vi "sortAndQueueLines.vi"(7 "scanning?":bool, 8 "error in (no error)":errorcluster, 11 "Queues":T2) -> (0 "error out":errorcluster, 1 "lost vol":cluster{"volume num":u32, "volume num":u32}[](array[cluster]), 3 "stats":T1, 5 "not waiting for new lines":bool)   [LabVIEW 2010]
uses:
  internal_queues.ctl
  line_info.ctl
  volume_with_lines.ctl
  volume_info.ctl
  kalman_result_scaled.ctl
  location3D.ctl
  spot location.ctl
  splitLinesIntoVolumes.vi
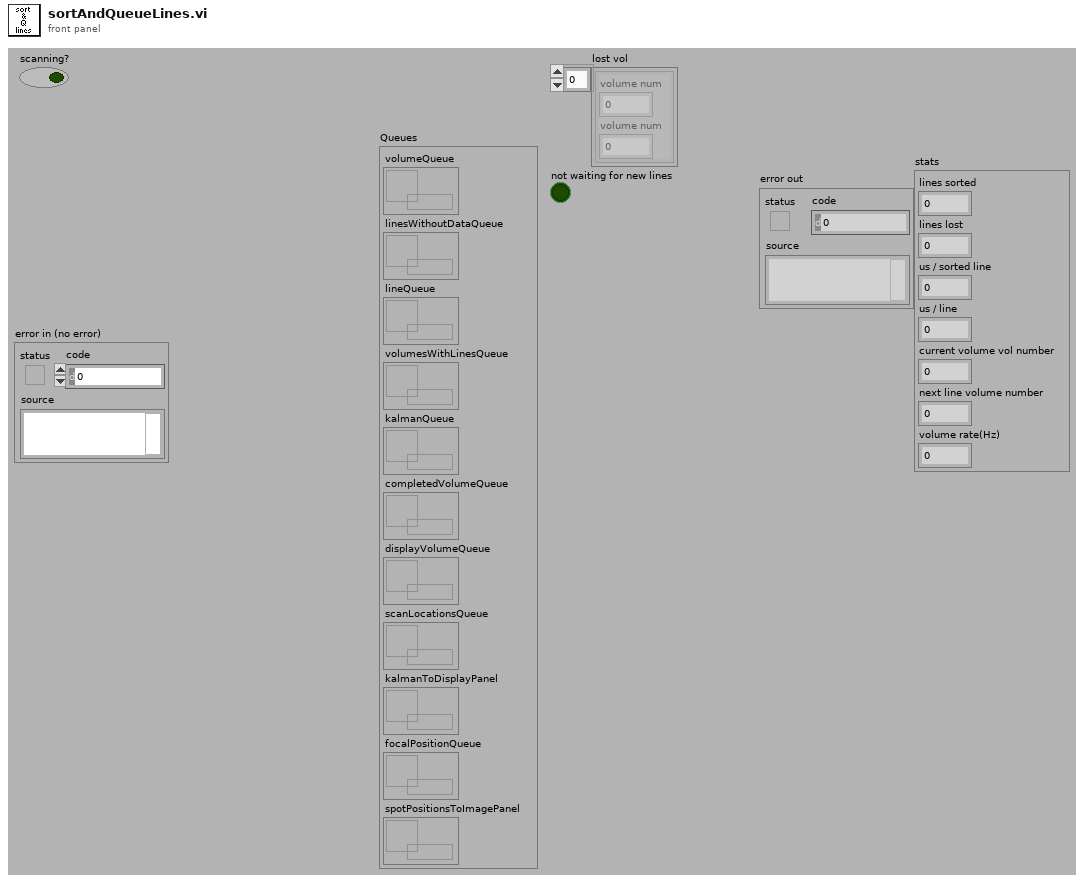
[diagram p1: front panel]
types:
  T1 = cluster{"lines sorted":i32, "lines lost":i32, "us / sorted line":dbl, "us / line":dbl, "current volume vol number":u32, "next line volume number":u32, "volume rate(Hz)":dbl}
  T2 = typedef "internal_queues.ctl" = cluster{"volumeQueue":refnum<queue>, "linesWithoutDataQueue":refnum<queue>, "lineQueue":refnum<queue>, "volumesWithLinesQueue":refnum<queue>, "kalmanQueue":refnum<queue>, "completedVolumeQueue":refnum<queue>, "displayVolumeQueue":refnum<queue>, "scanLocationsQueue":refnum<queue>, "kalmanToDisplayPanel":refnum<queue>, "focalPositionQueue":refnum<queue>, "spotPositionsToImagePanel":refnum<queue>}
  T3 = typedef "line_info.ctl" = cluster{"start X":i16, "start Y":i16, "start Z":i16, "end X":i16, "end Y":i16, "end Z":i16, "num z":u8, "voxel data":u32[], "volume num":u32, "line number":u16, "line type":u16}
  T4 = cluster{i32, i32, dbl, dbl, "last volume processed":u32, "volume num":u32, dbl}
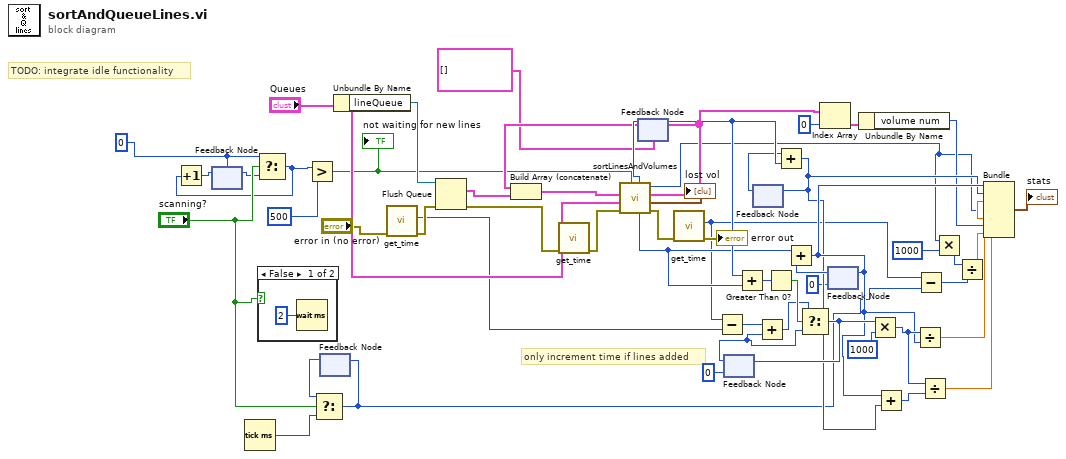
[diagram p0: block diagram]
diagram:
  w4 = u32 0 ("t")
  # "TODO: integrate idle functionality"
  # "only increment time if lines added"
  n1 = feedback #1(w4) -> (w5:u32)
  n2 = Tick Count (ms)() -> (millisecond timer value=w18:u32)
  n3 = Select(t=w4, s="scanning?", f=w5) -> (s? t:f=w3:u32)
  n4 = Increment(x=w3) -> (x+1=w6:u32)
  n5 = feedback-in #1(w6) -> ()
  n6 = case shown="False" "scanning?" {
    frame False {
      n7 = Wait (ms)(milliseconds to wait=u32 2) -> ()  [unwired: 1 out]
    }
    frame True {
    }
  }
  n8 = Greater?(x=w3, y=u32 500) -> (0:w1:bool)
  "not waiting for new lines" <- w1
  n9 = feedback #2() -> (w17:u32)  [unwired: 1 in]
  n10 = Select(t=w17, s="scanning?", f=w18) -> (s? t:f=w15:u32)
  n11 = feedback-in #2(w15) -> ()
  n12 = Unbundle By Name("Queues") -> ("lineQueue"=w54:refnum<queue>)
  n13 = call "get_time.vi"("error in (no error)"="error in (no error)") -> ("error out"=w49:errorcluster, "millisecond timer value"=w44:u32)  [unwired: 9 in]
  n14 = Flush Queue(queue=w54, error in (no error)=w49) -> (remaining elements=w53:T3[], error out=w48:errorcluster)  [unwired: 1 out]
  n15 = call "get_time.vi"("error in (no error)"=w48) -> ("error out"=w47:errorcluster)  [unwired: 9 in, 1 out]
  n16 = feedback #3(T3[] [] ("t")) -> (w20:T3[])
  n17 = Build Array (concatenate)(w20, w53) -> (w52:T3[])
  n18 = call "sortLinesAndVolumes.vi"("no new lines coming"=w1, "error in (no error)"=w47, "Queues"="Queues", "Array of lines"=w52) -> ("error out"=w46:errorcluster, "lost vol"=→"lost vol":cluster{"volume num":u32, "num lines":u32}[], "leftover lines"=w25:T3[], "last volume processed"=w8:u32, "lines sorted"=w40:i32, "lines lost"=w41:i32)  [unwired: 2 in]
  n19 = feedback-in #3(w25) -> ()
  n20 = call "get_time.vi"("error in (no error)"=w46) -> ("error out"=→"error out":errorcluster, "millisecond timer value"=w16:u32)  [unwired: 9 in]
  n21 = Subtract(x=w16, y=w44) -> (x-y=w43:u32)
  n22 = feedback #4(u32 0) -> (w36:u32)
  n23 = Add(x=w41, y=w40) -> (x+y=w39:i32)
  n24 = feedback #5() -> (w34:i32)  [unwired: 1 in]
  n25 = Add(x=w43, y=w36) -> (x+y=w35:u32)
  n26 = Greater Than 0?(x=w39) -> (x > 0?=w37:bool)
  n27 = Add(x=w34, y=w41) -> (x+y=w26:i32)
  n28 = feedback-in #5(w26) -> ()
  n29 = Select(t=w35, s=w37, f=w36) -> (s? t:f=w38:u32)
  n30 = feedback-in #4(w38) -> ()
  n31 = Index Array(array=w25, index=0) -> (element=w23:T3)
  n32 = feedback #6(0) -> (w33:i32)
  n33 = Add(x=w40, y=w33) -> (x+y=w27:i32)
  n34 = feedback-in #6(w27) -> ()
  n35 = Unbundle By Name(w23) -> ("volume num"=w13:u32)
  n36 = Multiply(x=w38, y=u32 1000) -> (x*y=w32:u32)
  n37 = Add(x=w27, y=w26) -> (x+y=w31:i32)
  n38 = Divide(x=w32, y=w27) -> (x/y=w30:dbl)
  n39 = Subtract(x=w16, y=w15) -> (x-y=w14:u32)
  n40 = Divide(x=w32, y=w31) -> (x/y=w29:dbl)
  n41 = Multiply(x=w8, y=u32 1000) -> (x*y=w11:u32)
  n42 = Divide(x=w11, y=w14) -> (x/y=w10:dbl)
  n43 = Bundle(w27, w26, w30, w29, "last volume processed"=w8, "volume num"=w13, w10) -> (→"stats":T4)  [unwired: 1 in]
